vi "ManualCommands.vi"() -> ()   [LabVIEW 2017, in "DemoSequencer.lvlib"]
uses:
  DemoSequencer.lvlib
  Utilities/StateMachine.ctl
  Utilities/Controlword_Commands.ctl
  Utilities/WordManipulationLibrary.lvlib
  Utilities/Bit Manipulation.lvlib
panel:
  in  "Clear Bit?":bool
  out "Enum":T1
  in  "set bit?":bool
  in  "Bit to set":u8
  in  "Device Control Command":T2
  in  "ControlWord In":u16 format="%08b"
  out "Status":T1
  out "StatusWord":u16 format="%08b"
  out "Results":dbl[](array[numeric])
  in  "Parameters":dbl[](array[numeric])
  in  "stop":bool
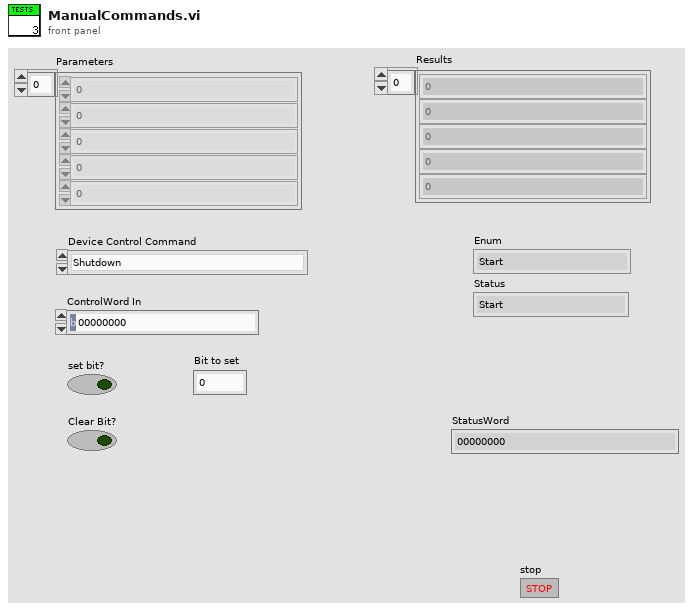
[diagram p1: front panel]
types:
  T1 = typedef "WordManipulationLibrary.lvlib/StateMachine.ctl" = enum16{"Start", "Not Ready to Switch On", "Switch On Disabled", "Ready to Switch On", "Switched On", "Operation enable", "Quick Stop Active", "Fault Reaction Active", "Fault"}
  T2 = typedef "WordManipulationLibrary.lvlib/Controlword_Commands.ctl" = enum16{"Shutdown", "Switch On", "Disable Voltage", "Quick Stop", "Disable Op", "Enable Op", "Fault Reset", "Error"}
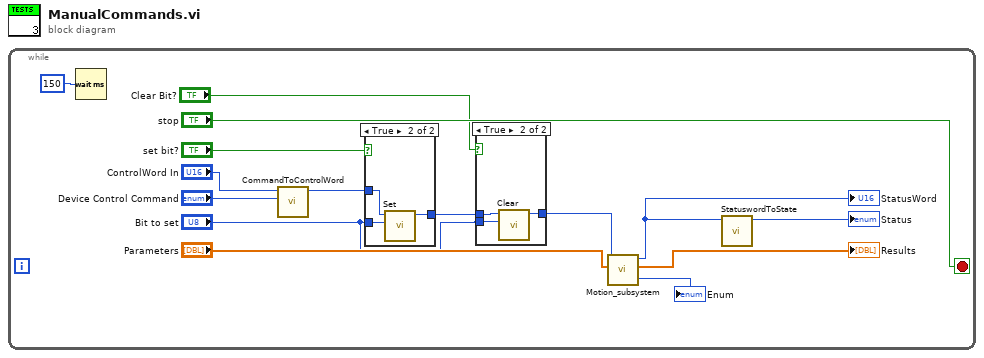
[diagram p0: block diagram]
diagram:
  n1 = while {
    stop <- "stop" stop-if-true
    n2 = Wait (ms)(milliseconds to wait=u32 150) -> ()  [unwired: 1 out]
    n3 = call "CommandToControlWord.vi"("Device Control Command"="Device Control Command", "ControlWord In"="ControlWord In") -> ("ControlWord Out"=w10:u16)  [unwired: 9 in]
    n4 = case shown="True" "set bit?" {
      tunnel: w10 -> [w20 w23]
      tunnel: [w20 w22] -> w4
      tunnel: "Bit to set" -> [_ w21]
      frame False {
      }
      frame True {
        n5 = call "Set.vi"("Bit to set"=w21, "Data_In"=w23) -> ("Data_Out"=w22:u16)  [unwired: 9 in]
      }
    }
    n6 = case shown="True" "Clear Bit?" {
      tunnel: w4 -> [w16 w18]
      tunnel: [w16 w19] -> w1
      tunnel: "Bit to set" -> [_ w17]
      frame False {
      }
      frame True {
        n7 = call "Clear.vi"("Bit to clear"=w17, "Data_In"=w18) -> ("Data_Out"=w19:u16)  [unwired: 9 in]
      }
    }
    n8 = call "Motion_subsystem.vi"("Parameters"="Parameters", "ControlWord"=w1) -> ("Results"=→"Results":dbl[], "StatusWord"=w6:u16, "Enum"=→"Enum":T1)  [unwired: 7 in]
    "StatusWord" <- w6
    n9 = call "StatuswordToState.vi"("Data_In"=w6) -> ("Status"=→"Status":T1)  [unwired: 10 in]
  }
